vi "Set Stop Trigger (Digital Edge).vi"(7 "Post-Trigger Duration (0 s)":dbl, 8 "error in (no error)":errorcluster, 9 "Trigger Channel":string, 10 "Slope":T1, 11 "Data Logging Specification Ref in":T2) -> (0 "error out":errorcluster, 3 "Data Logging Specification Ref out":T2)   [LabVIEW 2020, in "NI_VS Data Logging API.lvlib"]
doc: "Specifies a trigger condition on which to stop logging data. You also can specify whether to continue logging channel data for a set period of time after the trigger condition occurs.\n\nYou must manually select the polymorphic instance to use."
uses:
  <vilib>/NI VeriStand/Execution/DataLogging/NI_VS Data Logging API.lvlib
  <vilib>/NI VeriStand/Execution/DataLogging/DataLoggingSpecification Ref.ctl
  NationalInstruments.VeriStand.ClientAPI
  <vilib>/NI VeriStand/Execution/DataLogging/Slope.ctl
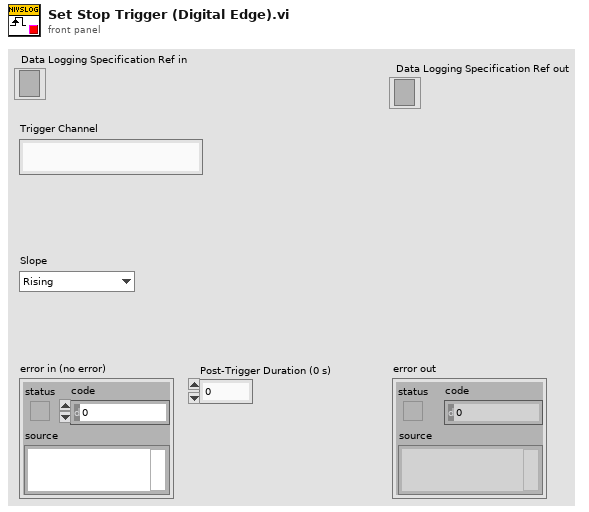
[diagram p1: front panel]
types:
  T1 = typedef "NI_VS Data Logging API.lvlib/Slope.ctl" = enum16{"Rising", "Falling"}
  T2 = typedef "NI_VS Data Logging API.lvlib/DataLoggingSpecification Ref.ctl" = refnum<k24>
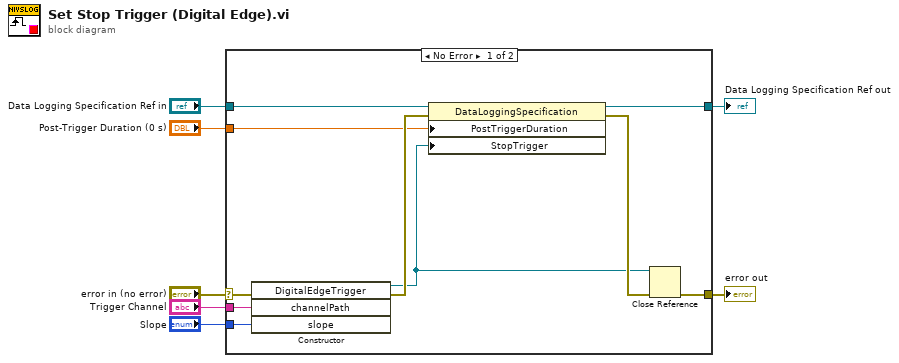
[diagram p0: block diagram]
diagram:
  n1 = case shown="No Error" "error in (no error)" {
    selector: "error in (no error)" -> [w14 w19]
    tunnel: "Trigger Channel" -> [w13 _]
    tunnel: "Data Logging Specification Ref in" -> [w15 w18]
    tunnel: [w10 w18] -> w5
    tunnel: [w9 w19] -> w4
    tunnel: "Post-Trigger Duration (0 s)" -> [w8 _]
    tunnel: "Slope" -> [w11 _]
    frame No Error {
      n2 = constructor class="DigitalEdgeTrigger"(error in=w14, "channelPath"=w13, "slope"=w11) -> (reference out=w12:refnum<k24>, error out=w17:errorcluster)  [unwired: 2 in, 3 out]
      n3 = property class="DataLoggingSpecification"(reference=w15, error in=w17, "PostTriggerDuration"=w8, "StopTrigger"=w12) -> (reference out=w10:T2, error out=w16:errorcluster)
      n4 = Close Reference(reference=w12, error in (no error)=w16) -> (error out=w9:errorcluster)
    }
    frame Error {
    }
  }
  "error out" <- w4
  "Data Logging Specification Ref out" <- w5
